vi "AngleScanInitializeAngles.vi"(9 "Step Size (deg)":dbl, 10 "Initial Angle (deg)":dbl, 11 "Final Angle (deg)":dbl) -> (2 "Angles (numeric)":dbl[](array[numeric]), 3 "Angles (string)":string[](array[string]))   [LabVIEW 2012]
panel:
  out "Angles":string[][](array[string])
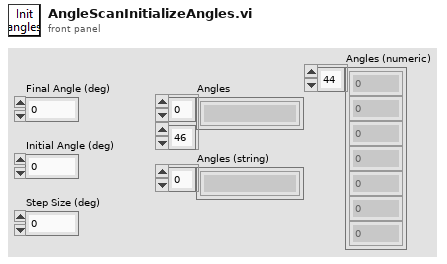
[diagram p1: front panel]
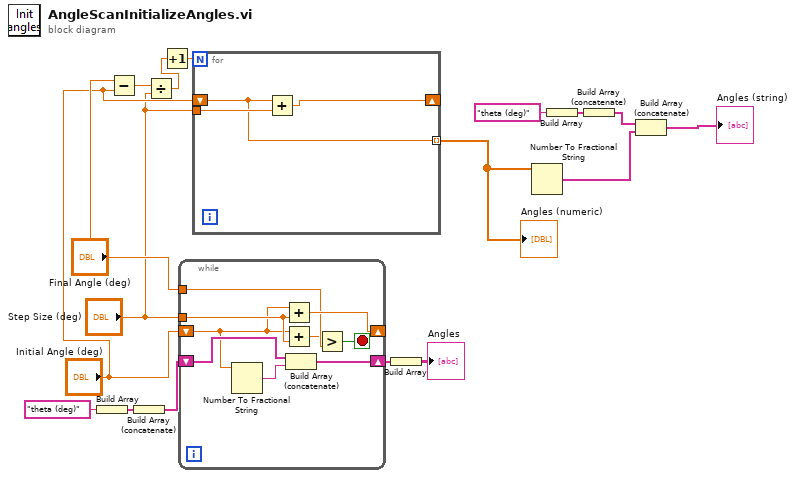
[diagram p0: block diagram]
diagram:
  n1 = Build Array("theta (deg)") -> (w15:string[])
  n2 = Subtract(x="Final Angle (deg)", y="Initial Angle (deg)") -> (x-y=w11:dbl)
  n3 = Build Array (concatenate)(w15) -> (w17:string[])
  n4 = Divide(x=w11, y="Step Size (deg)") -> (x/y=w1:dbl)
  n5 = Increment(x=w1) -> (x+1=w2:dbl)
  n6 = while {
    shift-right: [w22] -> _
    shift-left: "Initial Angle (deg)" -> [w18]
    tunnel: "Final Angle (deg)" -> [w21]
    shift-right: [w24] -> w14
    shift-left: w17 -> [w25]
    tunnel: "Step Size (deg)" -> [w20]
    stop <- w26 stop-if-true
    n7 = Number To Fractional String(number=w18) -> (F-format string=w23:string)  [unwired: 3 in]
    n8 = Add(x=w18, y=w20) -> (x+y=w22:dbl)
    n9 = Add(x=w18, y=w20) -> (x+y=w19:dbl)
    n10 = Build Array (concatenate)(w25, w23) -> (w24:string[])
    n11 = Greater?(x=w19, y=w21) -> (0:w26:bool)
  }
  n12 = for {
    N: w2 -> [_]
    tunnel: "Step Size (deg)" -> [w29]
    shift-right: [w28] -> _
    shift-left: "Initial Angle (deg)" -> [w27]
    tunnel: [w27] -> w8 mode=indexing
    n13 = Add(x=w27, y=w29) -> (x+y=w28:dbl)
  }
  "Angles (numeric)" <- w8
  n14 = Build Array(w14) -> (→"Angles":string[][])
  n15 = Number To Fractional String(number=w8) -> (F-format string=w4:string[])  [unwired: 3 in]
  n16 = Build Array("theta (deg)") -> (w7:string[])
  n17 = Build Array (concatenate)(w7) -> (w5:string[])
  n18 = Build Array (concatenate)(w5, w4) -> (→"Angles (string)":string[])
